vi "Collapsed Terminals.vi"(11 "State":T9) -> (3 "Terms":T1)   [LabVIEW 2020, in "Parallel Diagram Block.xnode"]
uses:
  Parallel Diagram Block.xnode
  State.ctl
  Parallel Block/Type Descriptor.ctl
  Parallel Block/Direction.ctl
  Parallel Block/Value Type.ctl
  Parallel Block/Terminal Mode.ctl
  <vilib>/picture/picture.llb/imagedata.ctl
  <vilib>/XNodeSupport/XNodeTerm4Array.ctl
  <vilib>/XNodeSupport/XNodeTerm4.ctl
  <vilib>/XNodeSupport/XNodeString.ctl
  <vilib>/XNodeSupport/XNodeVariant.ctl
  <vilib>/XNodeSupport/XNodeRect32.ctl
  <vilib>/XNodeSupport/XNodeInt.ctl
  <vilib>/XNodeSupport/XNodeBool.ctl
  <vilib>/XNodeSupport/XNodeTermDirection.ctl
  Parallel Block/Parallel Block.lvlib
  <vilib>/XNodeSupport/NI_XNodeSupport.lvlib
  Parallel Block/Terminal Type.ctl
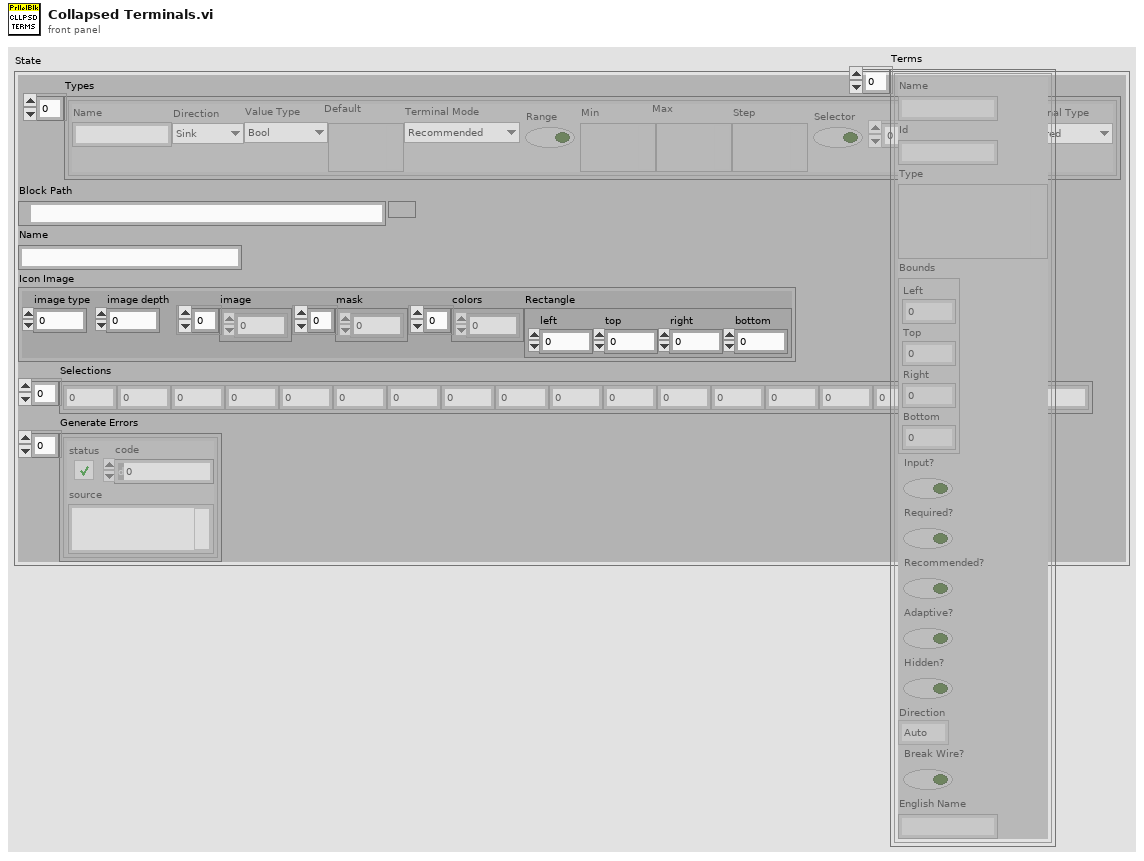
[diagram p1: front panel]
types:
  T1 = typedef "NI_XNodeSupport.lvlib/XNodeTerm4Array.ctl" = T2[]
  T2 = typedef "NI_XNodeSupport.lvlib/XNodeTerm4.ctl" = cluster{"Name":T3, "Id":T3, "Type":T4, "Bounds":T5, "Input?":T7, "Required?":T7, "Recommended?":T7, "Adaptive?":T7, "Hidden?":T7, "Direction":T8, "Break Wire?":T7, "English Name":T3}
  T3 = typedef "NI_XNodeSupport.lvlib/XNodeString.ctl" = string
  T4 = typedef "NI_XNodeSupport.lvlib/XNodeVariant.ctl" = variant
  T5 = typedef "NI_XNodeSupport.lvlib/XNodeRect32.ctl" = cluster{"Left":T6, "Top":T6, "Right":T6, "Bottom":T6}
  T6 = typedef "NI_XNodeSupport.lvlib/XNodeInt.ctl" = i32
  T7 = typedef "NI_XNodeSupport.lvlib/XNodeBool.ctl" = bool
  T8 = typedef "NI_XNodeSupport.lvlib/XNodeTermDirection.ctl" = enum32{"Auto", "Up", "Down", "Left", "Right", "Center"}
  T9 = typedef "Parallel Diagram Block.xnode/State.ctl" = cluster{"Types":T10[], "Block Path":path, "Name":string, "Icon Image":T15, "Selections":i32[], "Generate Errors":errorcluster[]}
  T10 = typedef "Parallel Block.lvlib/Type Descriptor.ctl" = cluster{"Name":string, "Direction":T11, "Value Type":T12, "Default":variant, "Terminal Mode":T13, "Range":bool, "Min":variant, "Max":variant, "Step":variant, "Selector":bool, "Options":string[], "Terminal Type":T14}
  T11 = typedef "Parallel Block.lvlib/Direction.ctl" = enum16{"Sink", "Source"}
  T12 = typedef "Parallel Block.lvlib/Value Type.ctl" = enum16{"Unknown", "Bool", "U8", "U16", "U32", "U64", "I8", "I16", "I32", "I64", "SGL", "DBL", "CSG", "CDB", "CDBWfm", "String", "DBLWfm"}
  T13 = typedef "Parallel Block.lvlib/Terminal Mode.ctl" = enum16{"Recommended", "Required", "None"}
  T14 = typedef "Parallel Block.lvlib/Terminal Type.ctl" = enum16{"Unwired", "BadType", "Connection", "Value", "Control Ref", "BadRefType"}
  T15 = typedef "imagedata.ctl" = cluster{"image type":i32, "image depth":i32, "image":u8[], "mask":u8[], "colors":u32[], "Rectangle":cluster{"left":i16, "top":i16, "right":i16, "bottom":i16}}
  T16 = cluster{"left":i16, "top":i16, "right":i16, "bottom":i16}
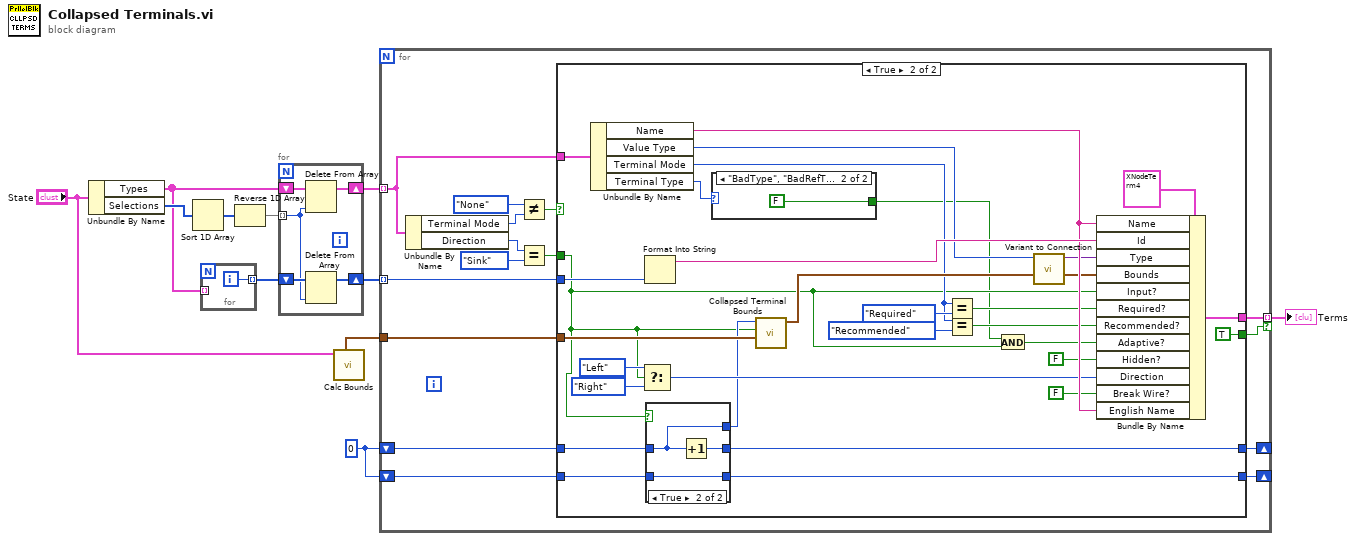
[diagram p0: block diagram]
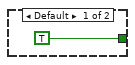
[diagram p3: hidden frame]
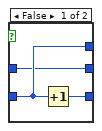
[diagram p4: hidden frame]
diagram:
  w1 = 0
  n1 = Unbundle By Name("State") -> ("Types"=w5:T10[], "Selections"=w9:i32[])
  n2 = Sort 1D Array(array=w9) -> (sorted array=w8:i32[])
  n3 = for {
    tunnel: w5 -> [_] mode=indexing
    tunnel: [w12] -> w4 mode=indexing
    i -> [w12]
  }
  n4 = Reverse 1D Array(array=w8) -> (reversed array=w7:i32[])
  n5 = for {
    tunnel: w7 -> [w13] mode=indexing
    shift-right: [w16] -> w6
    shift-left: w5 -> [w17]
    shift-right: [w14] -> w3
    shift-left: w4 -> [w15]
    n6 = Delete From Array(array=w17, index=w13) -> (array with subset deleted=w16:T10[])  [unwired: 1 in, 1 out]
    n7 = Delete From Array(array=w15, index=w13) -> (array with subset deleted=w14:i32[])  [unwired: 1 in, 1 out]
  }
  n8 = call "Calc Bounds.vi"("State"="State") -> ("Full Bounds"=w2:T16)  [unwired: 6 in, 4 out]
  n9 = for {
    tunnel: w6 -> [w28] mode=indexing
    tunnel: w2 -> [w30]
    tunnel: [w29] -> w10 mode=indexing if=w19
    tunnel: w3 -> [w27] mode=indexing
    shift-right: [w23] -> _
    shift-left: w1 -> [w26]
    shift-right: [w22] -> _
    shift-left: w1 -> [w24]
    n10 = Unbundle By Name(w28) -> ("Terminal Mode"=w21:T13, "Direction"=w31:T11)
    n11 = Not Equal?(x=Terminal_Mode."None", y=w21) -> (x != y?=w18:bool)
    n12 = Equal?(x=w31, y=Direction."Sink" ("x")) -> (x = y?=w25:bool)
    n13 = case shown="True" w18 {
      tunnel: w30 -> [_ w54]
      tunnel: [_ w52] -> w29
      tunnel: w28 -> [_ w46]
      tunnel: w27 -> [_ w45]
      tunnel: w26 -> [w34 w44]
      tunnel: w25 -> [_ w38]
      tunnel: w24 -> [w33 w43]
      tunnel: [w34 w42] -> w23
      tunnel: [w33 w41] -> w22
      tunnel: [_ TRUE] -> w19
      frame False {
      }
      frame True {
        n14 = Unbundle By Name(w46) -> ("Name"=w62:string, "Value Type"=w56:T12, "Terminal Mode"=w47:T13, "Terminal Type"=w37:T14)
        n15 = Select(t=XNodeTermDirection."Left" ("Direction"), s=w38, f=XNodeTermDirection."Right" ("Direction")) -> (s? t:f=w59:T8)
        n16 = Format Into String(w45) -> (resulting string=w63:string)  [unwired: 3 in, 1 out]
        n17 = case shown="True" w38 {
          tunnel: w44 -> [w67 w70]
          tunnel: w43 -> [w68 w71]
          tunnel: [w67 w72] -> w42
          tunnel: [w69 w71] -> w41
          tunnel: [w68 w70] -> w40
          frame False {
            n18 = Increment(x=w68) -> (x+1=w69:i32)
          }
          frame True {
            n19 = Increment(x=w70) -> (x+1=w72:i32)
          }
        }
        n20 = case shown="\"BadType\", \"BadRefType\"" w37 {
          tunnel: [TRUE FALSE] -> w35
          frame Default {
          }
          frame "BadType", "BadRefType" {
          }
        }
        n21 = call "Collapsed Terminal Bounds.vi"("Border Without Terminals"=w54, "Input"=w38, "Index"=w40) -> ("Bounds"=w53:T5)  [unwired: 8 in]
        n22 = Equal?(x=w47, y=Terminal_Mode."Required") -> (x = y?=w51:bool)
        n23 = Equal?(x=w47, y=Terminal_Mode."Recommended") -> (x = y?=w50:bool)
        n24 = And(x=w35, y=w38) -> (x .and. y?=w36:bool)
        n25 = call "Variant to Connection.vi"("Value Type"=w56) -> ("Connection Class"=w55:variant)  [unwired: 10 in]
        n26 = Bundle By Name(cluster=T2 {"Name"="", "Id"="", "Type"=variant, "Bounds"={"Left"=0, "Top"=0, "Right"=0, "Bottom"=0}, "Input?"=FALSE, "Required?"=FALSE, "Recommended?"=FALSE, "Adaptive?"=FALSE, "Hidden?"=FALSE, "Direction"=enum."Auto", "Break Wire?"=FALSE, "English Name"=""} ("Term 4"), "Name"=w62, "Id"=w63, "Type"=w55, "Bounds"=w53, "Input?"=w38, "Required?"=w51, "Recommended?"=w50, "Adaptive?"=w36, "Hidden?"=T7 FALSE, "Direction"=w59, "Break Wire?"=T7 FALSE, "English Name"=w62) -> (w52:T2)
      }
    }
  }
  "Terms" <- w10
